vi "Run and wait.vi"(8 "错误输入":errorcluster, 9 "Script":string, 10 "Script Name":string="TSB_Script", 11 "VISA资源名称":refnum<visa-resource-name>) -> (0 "错误输出":errorcluster, 3 "VISA资源名称输出":refnum<visa-resource-name>)   [LabVIEW 2020]
uses:
  Global variable.vi
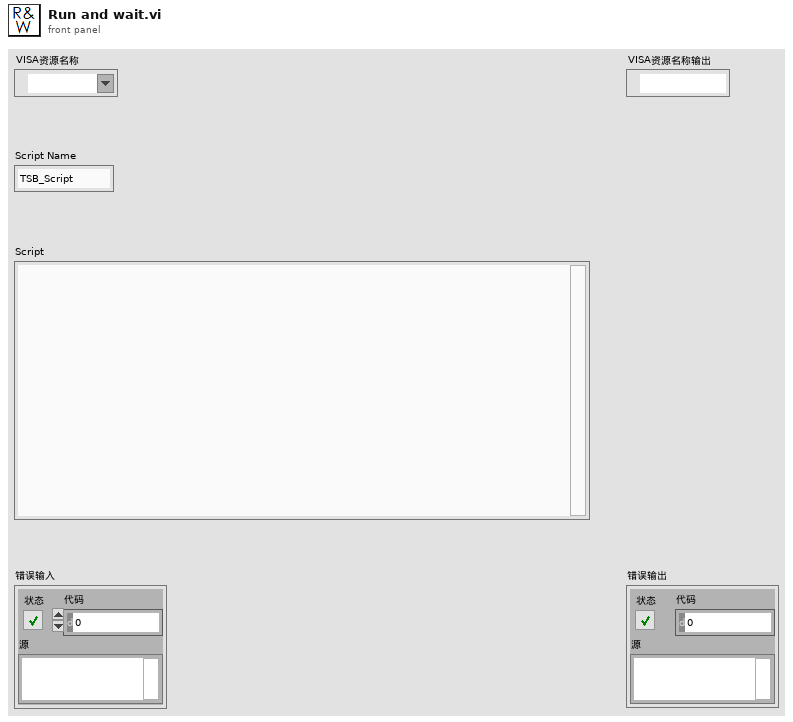
[diagram p1: front panel]
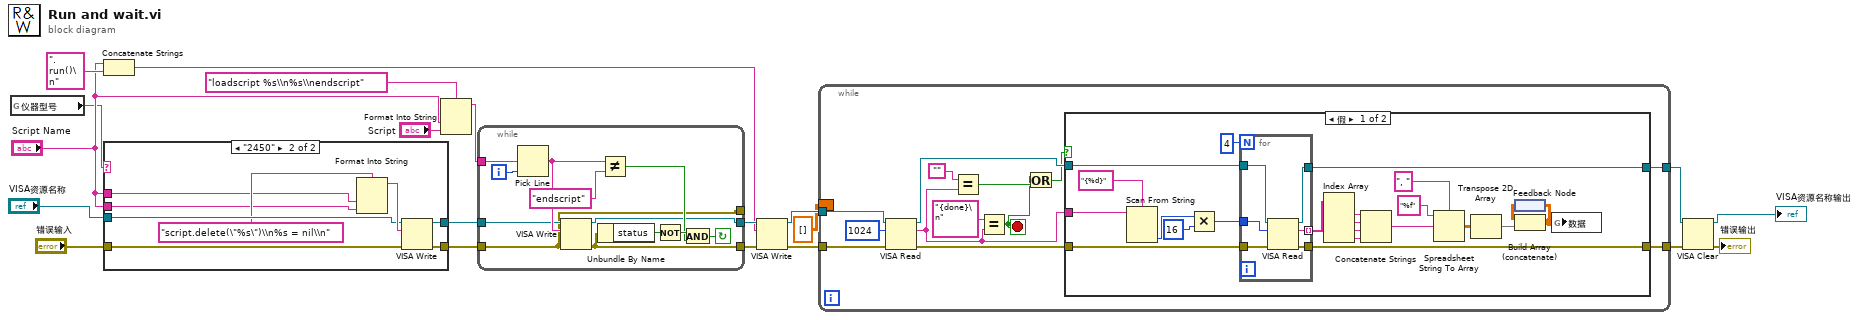
[diagram p0: block diagram]
diagram:
  n1 = global read "Global variable.vi" "仪器型号"() -> (w1:string)
  n2 = Concatenate Strings("Script Name", ".run()\n" ("string")) -> (w15:string)
  n3 = case shown="\"2450\"" w1 {
    tunnel: "错误输入" -> [w21 w29]
    tunnel: "VISA资源名称" -> [w22 w28]
    tunnel: "Script Name" -> [_ w26]
    tunnel: "Script Name" -> [_ w25]
    tunnel: [w21 w24] -> w3
    tunnel: [w22 w23] -> w2
    frame "2601B", Default {
    }
    frame "2450" {
      n4 = Format Into String(format string="script.delete(\"%s\")\\n%s = nil\\n", w26, w25) -> (resulting string=w30:string)  [unwired: 2 in, 1 out]
      n5 = VISA Write(VISA resource name=w28, write buffer=w30, error in (no error)=w29) -> (VISA resource name out=w23:refnum<visa-resource-name>, error out=w24:errorcluster)  [unwired: 1 out]
    }
  }
  n6 = Format Into String(format string="loadscript %s\\n%s\\nendscript", "Script Name", "Script") -> (resulting string=w19:string)  [unwired: 2 in, 1 out]
  n7 = while {
    tunnel: w19 -> [w41]
    tunnel: w2 -> [w34]
    tunnel: [w31] -> _
    tunnel: [w33] -> w18
    tunnel: [w32] -> w17
    tunnel: w3 -> [w31]
    i -> [w42]
    stop <- w35 continue-if-true
    n8 = Pick Line(multi-line string=w41, line index=w42) -> (output string=w39:string)  [unwired: 1 in]
    n9 = VISA Write(VISA resource name=w34, write buffer=w39, error in (no error)=w31) -> (VISA resource name out=w32:refnum<visa-resource-name>, error out=w33:errorcluster)  [unwired: 1 out]
    n10 = Unbundle By Name(w33) -> ("status"=w38:bool)
    n11 = Not Equal?(x=w39, y="endscript") -> (x != y?=w36:bool)
    n12 = Not(x=w38) -> (.not. x?=w37:bool)
    n13 = And(x=w37, y=w36) -> (x .and. y?=w35:bool)
  }
  n14 = VISA Write(VISA resource name=w17, write buffer=w15, error in (no error)=w18) -> (VISA resource name out=w12:refnum<visa-resource-name>, error out=w11:errorcluster)  [unwired: 1 out]
  n15 = while {
    tunnel: w12 -> [w54]
    tunnel: w11 -> [w53]
    tunnel: [w51] -> w9
    tunnel: [w50] -> w10
    border: dbl[][] [] -> [_]
    stop <- w43 stop-if-true
    n16 = VISA Read(VISA resource name=w54, byte count=u32 1024 ("字节总数"), error in (no error)=w53) -> (VISA resource name out=w49:refnum<visa-resource-name>, read buffer=w47:string, error out=w52:errorcluster)  [unwired: 1 out]
    n17 = Equal?(x="", y=w47) -> (x = y?=w44:bool)
    n18 = Equal?(x="{done}\n" ("y"), y=w47) -> (x = y?=w43:bool)
    n19 = Or(x=w43, y=w44) -> (x .or. y?=w45:bool)
    n20 = case shown="假" w45 {
      tunnel: w47 -> [w77 _]
      tunnel: w52 -> [w75 w84]
      tunnel: [w74 w84] -> w51
      tunnel: [w73 w85] -> w50
      tunnel: w49 -> [w72 w85]
      frame False {
        n21 = Scan From String(format string="{%d}" ("格式字符串"), input string=w77) -> (output 1=w70:i32)  [unwired: 3 in, 3 out]
        n22 = Multiply(x=w70, y=16) -> (x*y=w68:i32)
        n23 = for {
          N: 4 -> [_]
          tunnel: w75 -> [w83]
          tunnel: [w82] -> w74
          tunnel: [w81] -> w73
          tunnel: w72 -> [w80]
          tunnel: w68 -> [w79]
          tunnel: [w78] -> w62 mode=indexing
          n24 = VISA Read(VISA resource name=w80, byte count=w79, error in (no error)=w83) -> (VISA resource name out=w81:refnum<visa-resource-name>, read buffer=w78:string, error out=w82:errorcluster)  [unwired: 1 out]
        }
        n25 = Index Array(array=w62) -> (element #1=w61:string, element #2=w60:string, element #3=w59:string, element #4=w56:string)  [unwired: 4 in]
        n26 = Concatenate Strings(w61, w60, w59, w56) -> (w67:string)
        n27 = Spreadsheet String To Array(delimiter (Tab)=", " ("分隔符(Tab)"), format string="%f" ("格式字符串"), spreadsheet string=w67) -> (array=w64:dbl[][])  [unwired: 1 in]
        n28 = Transpose 2D Array(2D array=w64) -> (transposed array=w63:dbl[][])
        n29 = feedback #1() -> (w58:dbl[][])
        n30 = Build Array (concatenate)(w58, w63) -> (w57:dbl[][])
        n31 = feedback-in #1(w57) -> ()
        n32 = global write "Global variable.vi" "数据"(w57) -> ()
      }
      frame True {
      }
    }
  }
  n33 = VISA Clear(VISA resource name=w10, error in (no error)=w9) -> (VISA resource name out=→"VISA资源名称输出":refnum<visa-resource-name>, error out=→"错误输出":errorcluster)
